vi "K_grating.vi"(2 "error in (no error)":errorcluster, 3 "Grating, gr/mm":u16(ring)=2 items=["2400", "1800", "1200", "600", "300", "150"]) -> (0 "error out":errorcluster, 1 "K_grating":i16)   [LabVIEW 2018]
doc: "grating gr conversion to number"
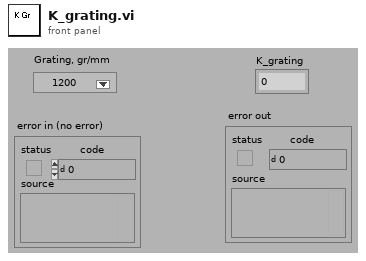
[diagram p1: front panel]
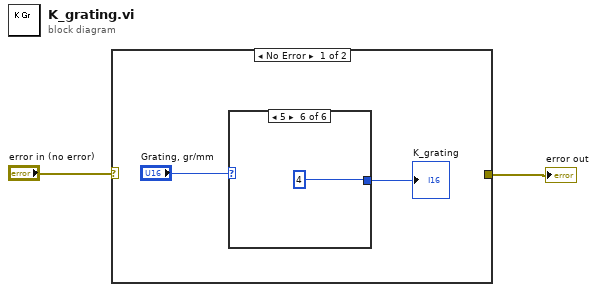
[diagram p0: block diagram]
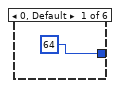
[diagram p2: hidden frame]
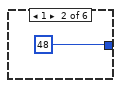
[diagram p3: hidden frame]
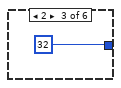
[diagram p4: hidden frame]
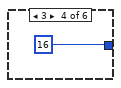
[diagram p5: hidden frame]
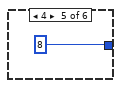
[diagram p6: hidden frame]
diagram:
  n1 = case shown="No Error" "error in (no error)" {
    selector: "error in (no error)" -> [_ w11]
    tunnel: [_ w11] -> w2
    frame No Error {
      n2 = case shown="5" "Grating, gr/mm" {
        tunnel: [64 48 32 16 8 4] -> w3
        frame 0, Default {
        }
        frame 1 {
        }
        frame 2 {
        }
        frame 3 {
        }
        frame 4 {
        }
        frame 5 {
        }
      }
      "K_grating" <- w3
    }
    frame Error {
    }
  }
  "error out" <- w2
